vi "OSC_Calc.vi"(8 "Flow":dbl, 9 "Lambda 2 Array":dbl[](array[numeric]), 10 "Lambda 1 Array":dbl[](array[numeric]), 11 "MFC":dbl) -> (1 "OSC-Meas Flow":dbl, 2 "OSC- Calc Flow":dbl, 3 "Calculated Flow":dbl)   [LabVIEW 2014]
uses:
  <vilib>/Analysis/baseanly.llb/Mean (DBL).vi
  <vilib>/Analysis/NI_AALPro.lvlib
  <vilib>/Analysis/NI_AALBase.lvlib
panel:
  out "L2 Avg Signal":dbl[](graph)
  out "Time":dbl
  out "mean":dbl format="%0.2f"
  out "mean 2":dbl format="%0.2f"
  out "mean 3":dbl format="%0.2f"
  out "L1 Gradient":dbl[](graph)
  out "L1 Avg Gradient":dbl[](graph)
  out "L1 Data":dbl[](graph)
  out "L1 Max Grad":dbl
  out "L1 TP":i32
  out "L2 Gradient":dbl[](graph)
  out "L2 Avg Gradient":dbl[](graph)
  out "L2 Data":dbl[](graph)
  out "L2 Max Grad":dbl
  out "L2 TP":i32
  # "OSC Calculation"
  # "Inputs"
  # "Outputs"
  # "Indicators"
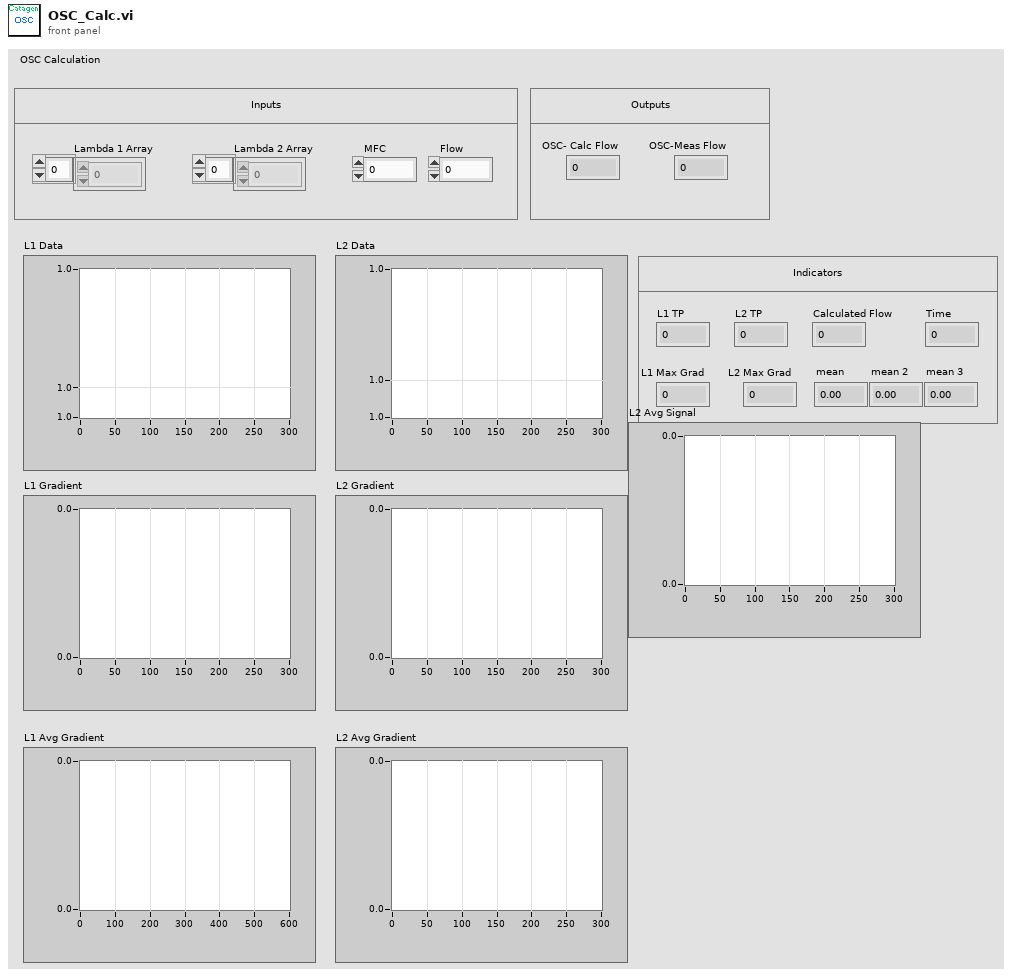
[diagram p1: front panel]
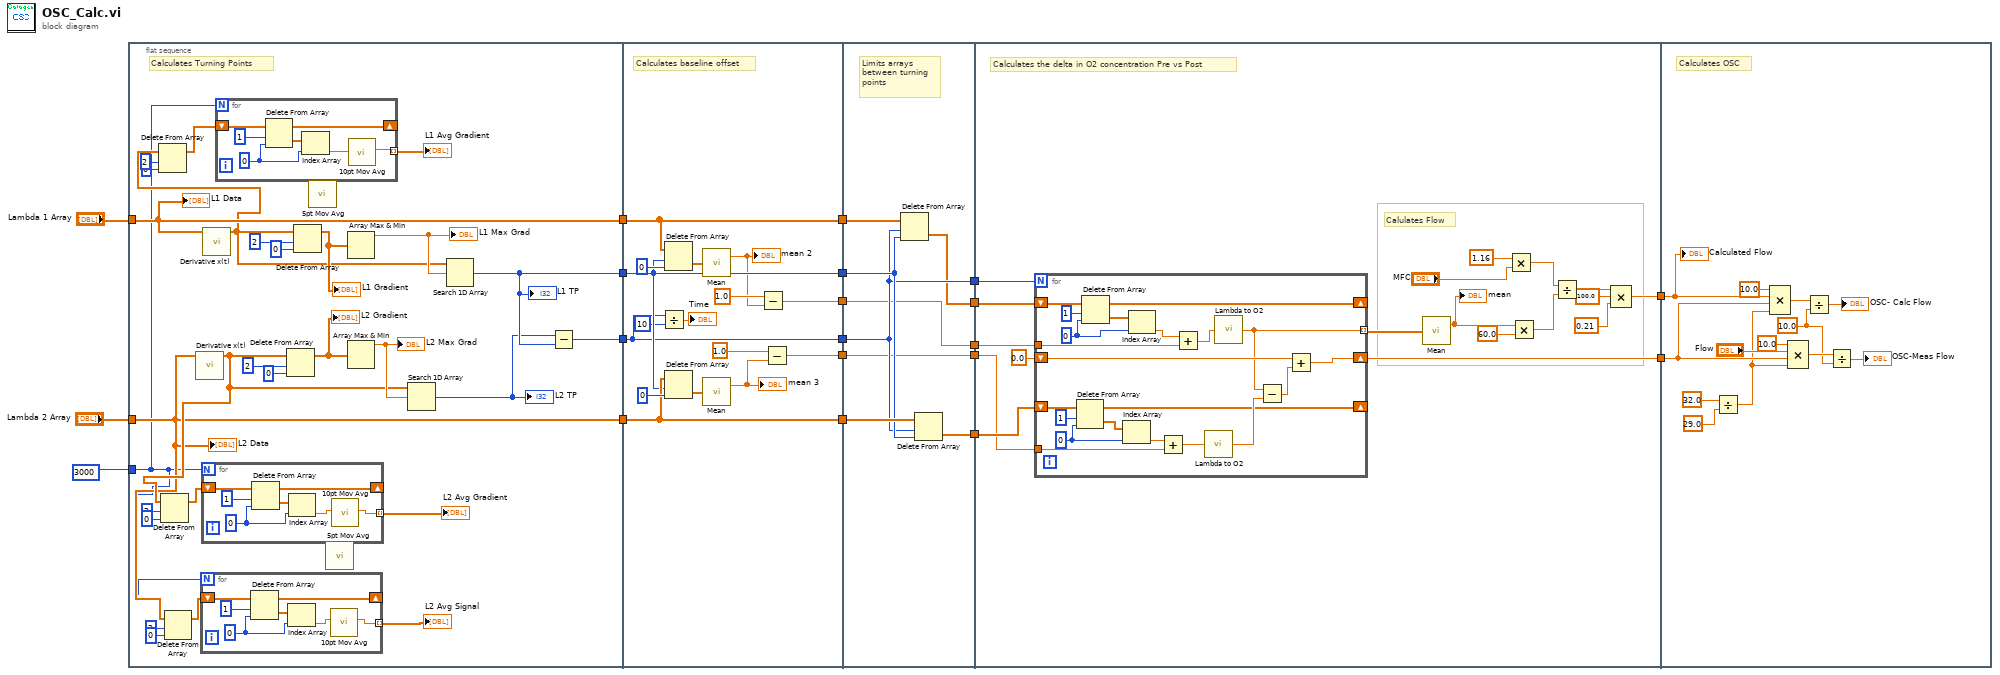
[diagram p0: block diagram]
diagram:
  n1 = flat-sequence {
    tunnel: [w24] -> w20
    tunnel: [w37] -> w19
    tunnel: [w42] -> w18
    tunnel: [w41] -> w17
    tunnel: "Lambda 1 Array" -> [w37]
    tunnel: "Lambda 2 Array" -> [w24]
    tunnel: 3000 -> [w21]
    tunnel: w20 -> [w80]
    tunnel: [w80] -> w16
    tunnel: w19 -> [w85]
    tunnel: [w85] -> w15
    tunnel: w18 -> [w72]
    tunnel: [w72] -> w14
    tunnel: w17 -> [w79]
    tunnel: [w79] -> w13
    tunnel: [w77] -> w12
    tunnel: [w73] -> w2
    tunnel: w16 -> [w92]
    tunnel: w15 -> [w93]
    tunnel: w14 -> [w90]
    tunnel: w13 -> [w91]
    tunnel: [w90] -> w11
    tunnel: [w89] -> w10
    tunnel: [w88] -> w9
    tunnel: w12 -> [w87]
    tunnel: [w87] -> w8
    tunnel: w2 -> [w86]
    tunnel: [w86] -> w1
    tunnel: w11 -> [w111]
    tunnel: w10 -> [w109]
    tunnel: w9 -> [w110]
    tunnel: [w107] -> w7
    tunnel: [w96] -> w6
    tunnel: w8 -> [w95]
    tunnel: w1 -> [w94]
    tunnel: w7 -> [w140]
    tunnel: w6 -> [w144]
    frame #0 {
      # "Calculates Turning Points"
      n2 = Delete From Array(array=w24, length=2, index=0) -> (array with subset deleted=w23:dbl[])  [unwired: 1 out]
      n3 = call <vilib>:"Derivative x(t).vi"("X"=w24) -> ("dX/dt"=w32:dbl[])  [unwired: 9 in, 1 out]
      n4 = Delete From Array(array=w32, length=2, index=0) -> (array with subset deleted=w31:dbl[])  [unwired: 1 out]
      n5 = for {
        N: w21 -> [_]
        tunnel: [w49] -> w22 mode=indexing
        shift-right: [w54] -> _
        shift-left: w23 -> [w53]
        w51 = 0 ("index")
        n6 = Delete From Array(array=w53, length=1, index=w51) -> (deleted portion=w52:dbl[], array with subset deleted=w54:dbl[])
        n7 = Index Array(array=w52, index=w51) -> (element=w50:dbl)
        n8 = call "10pt Mov Avg.vi"("Value in"=w50) -> ("Value out"=w49:dbl)  [unwired: 10 in]
      }
      "L2 Avg Signal" <- w22
      n9 = for {
        N: w21 -> [_]
        tunnel: [w56] -> w36 mode=indexing
        shift-right: [w61] -> _
        shift-left: w31 -> [w60]
        w58 = 0 ("index")
        n10 = Delete From Array(array=w60, length=1, index=w58) -> (deleted portion=w59:dbl[], array with subset deleted=w61:dbl[])
        n11 = Index Array(array=w59, index=w58) -> (element=w57:dbl)
        n12 = call "10pt Mov Avg.vi"("Value in"=w57) -> ("Value out"=w56:dbl)  [unwired: 10 in]
      }
      "L2 Avg Gradient" <- w36
      n13 = call <vilib>:"Derivative x(t).vi"("X"=w37) -> ("dX/dt"=w30:dbl[])  [unwired: 9 in, 1 out]
      n14 = Delete From Array(array=w30, length=2, index=0) -> (array with subset deleted=w29:dbl[])  [unwired: 1 out]
      n15 = for {
        N: w21 -> [_]
        tunnel: [w63] -> w35 mode=indexing
        shift-right: [w68] -> _
        shift-left: w29 -> [w67]
        w65 = 0 ("index")
        n16 = Delete From Array(array=w67, length=1, index=w65) -> (deleted portion=w66:dbl[], array with subset deleted=w68:dbl[])
        n17 = Index Array(array=w66, index=w65) -> (element=w64:dbl)
        n18 = call "10pt Mov Avg.vi"("Value in"=w64) -> ("Value out"=w63:dbl)  [unwired: 10 in]
      }
      "L1 Avg Gradient" <- w35
      n19 = Delete From Array(array=w32, length=2, index=0) -> (array with subset deleted=w39:dbl[])  [unwired: 1 out]
      "L2 Gradient" <- w39
      n20 = Delete From Array(array=w30, length=2, index=0) -> (array with subset deleted=w40:dbl[])  [unwired: 1 out]
      "L1 Gradient" <- w40
      n21 = call "5pt Mov Avg.vi"() -> ()  [unwired: 11 in, 1 out]
      n22 = call "5pt Mov Avg.vi"() -> ()  [unwired: 11 in, 1 out]
      n23 = Array Max & Min(array=w40) -> (max value=w46:dbl)  [unwired: 3 out]
      "L1 Max Grad" <- w46
      n24 = Array Max & Min(array=w39) -> (max value=w45:dbl)  [unwired: 3 out]
      "L2 Max Grad" <- w45
      n25 = Search 1D Array(1D array=w32, element=w45) -> (index of element=w38:i32)  [unwired: 1 in]
      "L2 TP" <- w38
      n26 = Search 1D Array(1D array=w30, element=w46) -> (index of element=w41:i32)  [unwired: 1 in]
      "L1 TP" <- w41
      n27 = Subtract(x=w38, y=w41) -> (x-y=w42:i32)
      "L1 Data" <- w37
      "L2 Data" <- w24
    }
    frame #1 {
      # "Calculates baseline offset"
      n28 = Divide(x=w72, y=10) -> (x/y=→"Time":dbl)
      n29 = Delete From Array(array=w85, length=w79, index=0) -> (deleted portion=w83:dbl[])  [unwired: 1 out]
      n30 = Delete From Array(array=w80, length=w79, index=0) -> (deleted portion=w82:dbl[])  [unwired: 1 out]
      n31 = call-poly <vilib>:"Mean.vi"("X"=w83) -> ("mean"=w75:dbl)  [unwired: 1 out]
      "mean 2" <- w75
      n32 = call-poly <vilib>:"Mean.vi"("X"=w82) -> ("mean"=w78:dbl)  [unwired: 1 out]
      "mean 3" <- w78
      n33 = Subtract(x=1.0, y=w75) -> (x-y=w73:dbl)
      n34 = Subtract(x=1.0, y=w78) -> (x-y=w77:dbl)
    }
    frame #2 {
      # "Limits arrays\nbetween turning\npoints"
      n35 = Delete From Array(array=w93, length=w90, index=w91) -> (deleted portion=w88:dbl[])  [unwired: 1 out]
      n36 = Delete From Array(array=w92, length=w90, index=w91) -> (deleted portion=w89:dbl[])  [unwired: 1 out]
    }
    frame #3 {
      # "Calculates the delta in O2 concentration Pre vs Post"
      # "Calulates Flow"
      n37 = for {
        N: w111 -> [_]
        shift-right: [w119] -> _
        shift-left: w110 -> [w132]
        shift-right: [w118] -> _
        shift-left: w109 -> [w125]
        shift-right: [w123] -> w107
        shift-left: 0.0 ("element") -> [w124]
        tunnel: [w120] -> w106 mode=indexing
        tunnel: w95 -> [w116]
        tunnel: w94 -> [w113]
        w128 = 0 ("index")
        w129 = 0 ("index")
        n38 = Delete From Array(array=w125, length=1, index=w128) -> (deleted portion=w127:dbl[], array with subset deleted=w118:dbl[])
        n39 = Delete From Array(array=w132, length=1, index=w129) -> (deleted portion=w130:dbl[], array with subset deleted=w119:dbl[])
        n40 = Index Array(array=w127, index=w128) -> (element=w117:dbl)
        n41 = Index Array(array=w130, index=w129) -> (element=w114:dbl)
        n42 = Add(x=w117, y=w116) -> (x+y=w115:dbl)
        n43 = Add(x=w114, y=w113) -> (x+y=w112:dbl)
        n44 = call "Lambda to O2.vi"("Lambda"=w115) -> ("O2 %"=w121:sgl)
        n45 = call "Lambda to O2.vi"("Lambda"=w112) -> ("O2 %"=w120:sgl)
        n46 = Subtract(x=w120, y=w121) -> (x-y=w122:sgl)
        n47 = Add(x=w124, y=w122) -> (x+y=w123:dbl)
      }
      n48 = call-poly <vilib>:"Mean.vi"("X"=w106) -> ("mean"=w103:dbl)  [unwired: 1 out]
      "mean" <- w103
      n49 = Multiply(x=1.16, y="MFC") -> (x*y=w101:dbl)
      n50 = Multiply(x=w103, y=60.0) -> (x*y=w100:dbl)
      n51 = Divide(x=w101, y=w100) -> (x/y=w99:dbl)
      n52 = Compound Arithmetic op=MULTIPLY(w99, 100.0 ("value"), 0.21 ("value")) -> (w96:dbl)
    }
    frame #4 {
      w133 = 10.0 ("y")
      # "Calculates OSC"
      n53 = Divide(x=32.0, y=29.0) -> (x/y=w138:dbl)
      n54 = Compound Arithmetic op=MULTIPLY(10.0 ("value"), w144, w140, w138) -> (w134:dbl)
      n55 = Compound Arithmetic op=MULTIPLY(10.0 ("value"), "Flow", w140, w138) -> (w135:dbl)
      n56 = Divide(x=w134, y=w133) -> (x/y=→"OSC- Calc Flow":dbl)
      n57 = Divide(x=w135, y=w133) -> (x/y=→"OSC-Meas Flow":dbl)
      "Calculated Flow" <- w144
    }
  }
